vi "SetRandomStrings.vi"(8 "error in (no error)":errorcluster, 11 "Snake in":refnum<class "SnakeGame.lvclass">) -> (0 "error out":errorcluster, 3 "Snake out":refnum<class "SnakeGame.lvclass">)   [LabVIEW 2019, in "RT_Game.lvlib" / "SnakeGame.lvclass"]
uses:
  SnakeGame.lvclass
  SnakeGame.lvclass/SnakeGame.ctl
  Game/Coordinate.ctl
  Game/Game.lvclass
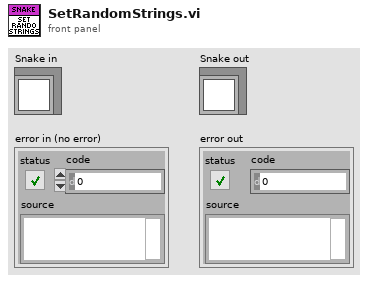
[diagram p1: front panel]
types:
  T1 = typedef "RT_Game.lvlib/Game.lvclass/Coordinate.ctl" = cluster{"x":i16, "y":i16}
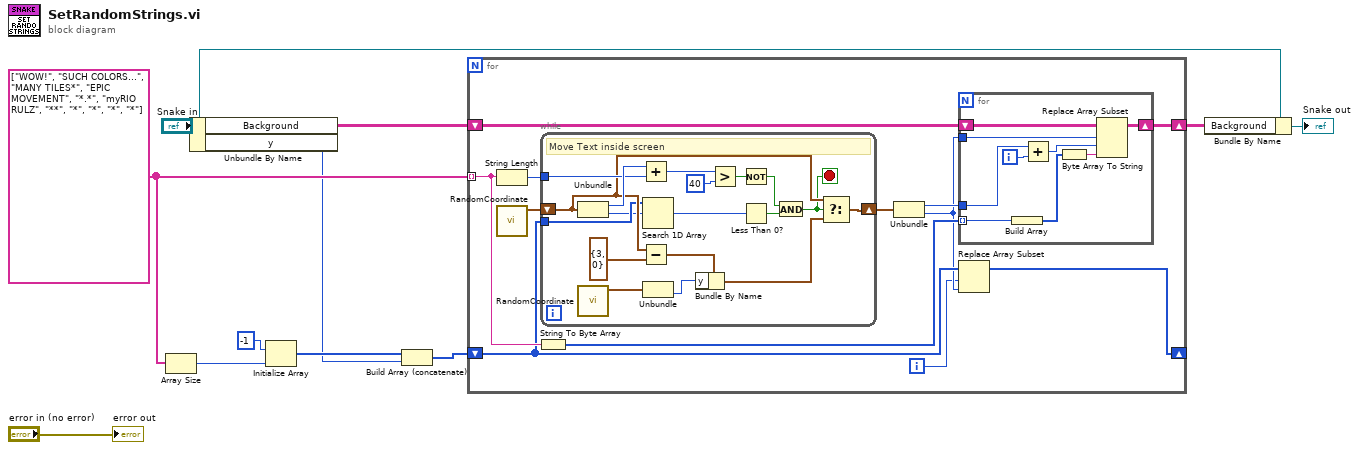
[diagram p0: block diagram]
diagram:
  w5 = string[] ["WOW!", "SUCH COLORS...", "MANY TILES*", "EPIC MOVEMENT", "*.*", "myRIO RULZ", "**", "*", "*", "*", "*"] ("String")
  n1 = Array Size(array=w5) -> (size(s)=w4:i32)
  n2 = Unbundle By Name("Snake in") -> ("Background"=w11:string[][], "y"=w1:i16)
  n3 = Initialize Array(-1 ("y_values"), w4) -> (w3:i32[])
  n4 = Build Array (concatenate)(w3, w1) -> (w2:i32[])
  n5 = for {
    shift-right: [w20] -> w7
    shift-left: w11 -> [w23]
    tunnel: w5 -> [w19] mode=indexing
    shift-right: [w15] -> _
    shift-left: w2 -> [w14]
    i -> [w12]
    n6 = String Length(string=w19) -> (length=w18:i32)
    n7 = call "RandomCoordinate.vi"() -> ("Coordinate"=w17:T1)  [unwired: 11 in]
    n8 = String To Byte Array(string=w19) -> (unsigned byte array=w21:u8[])
    n9 = while {
      tunnel: w18 -> [w40]
      shift-right: [w35] -> w16
      shift-left: w17 -> [w34]
      tunnel: w14 -> [w31]
      stop <- w24 stop-if-true
      # "Move Text inside screen"
      n10 = Unbundle(w34) -> ("x"=w41:i16, "y"=w25:i16)
      n11 = call "RandomCoordinate.vi"() -> ("Coordinate"=w29:T1)  [unwired: 11 in]
      n12 = Add(x=w41, y=w40) -> (x+y=w39:i32)
      n13 = Subtract(x=w34, y=T1 {"x"=3, "y"=0}) -> (x-y=w32:T1)
      n14 = Search 1D Array(1D array=w31, element=w25) -> (index of element=w28:i32)  [unwired: 1 in]
      n15 = Unbundle(w29) -> ("y"=w26:i16)  [unwired: 1 out]
      n16 = Bundle By Name(cluster=w32, "y"=w26) -> (w30:T1)
      n17 = Greater?(x=w39, y=40) -> (0:w36:bool)
      n18 = Not(x=w36) -> (.not. x?=w37:bool)
      n19 = Less Than 0?(x=w28) -> (x < 0?=w27:bool)
      n20 = And(x=w37, y=w27) -> (x .and. y?=w24:bool)
      n21 = Select(t=w34, s=w24, f=w30) -> (s? t:f=w35:T1)
    }
    n22 = Unbundle(w16) -> ("x"=w22:i16, "y"=w13:i16)
    n23 = for {
      tunnel: w13 -> [w49]
      tunnel: w22 -> [w48]
      shift-right: [w45] -> w20
      shift-left: w23 -> [w50]
      tunnel: w21 -> [w44] mode=indexing
      i -> [w46]
      n24 = Build Array(w44) -> (w42:u8[])
      n25 = Add(x=w48, y=w46) -> (x+y=w47:i32)
      n26 = Byte Array To String(unsigned byte array=w42) -> (string=w43:string)
      n27 = Replace Array Subset(array=w50, new element=w43, index (row)=w49, index (col)=w47) -> (w45:string[][])
    }
    n28 = Replace Array Subset(array=w14, new element=w13, index=w12) -> (w15:i32[])
  }
  n29 = Bundle By Name(cluster="Snake in", "Background"=w7) -> (→"Snake out":refnum<class "SnakeGame.lvclass">)
  "error out" <- "error in (no error)"
